vi "UI메시지전달.vi"() -> ()   [LabVIEW 2014]
panel:
  out "에러 출력":errorcluster
  in  "Configuration":T1
  in  "정지":bool
  in  "Stop Control":bool
  in  "Start Control":bool
  in  "Update Configuration":bool
  in  "Connect":bool
  out "메시지 출력":string
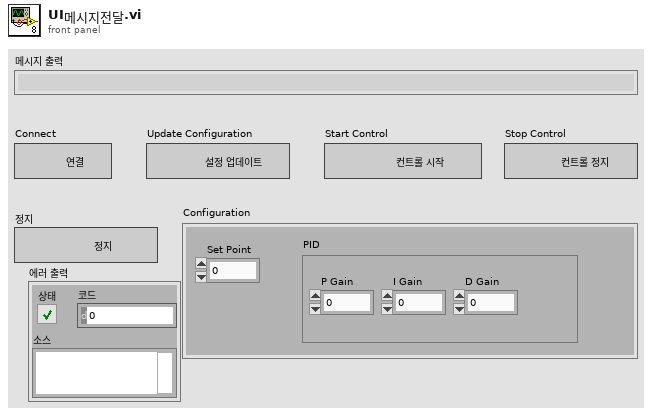
[diagram p1: front panel]
types:
  T1 = cluster{"Set Point":dbl, "PID":cluster{"P Gain":dbl, "I Gain":dbl, "D Gain":dbl}}
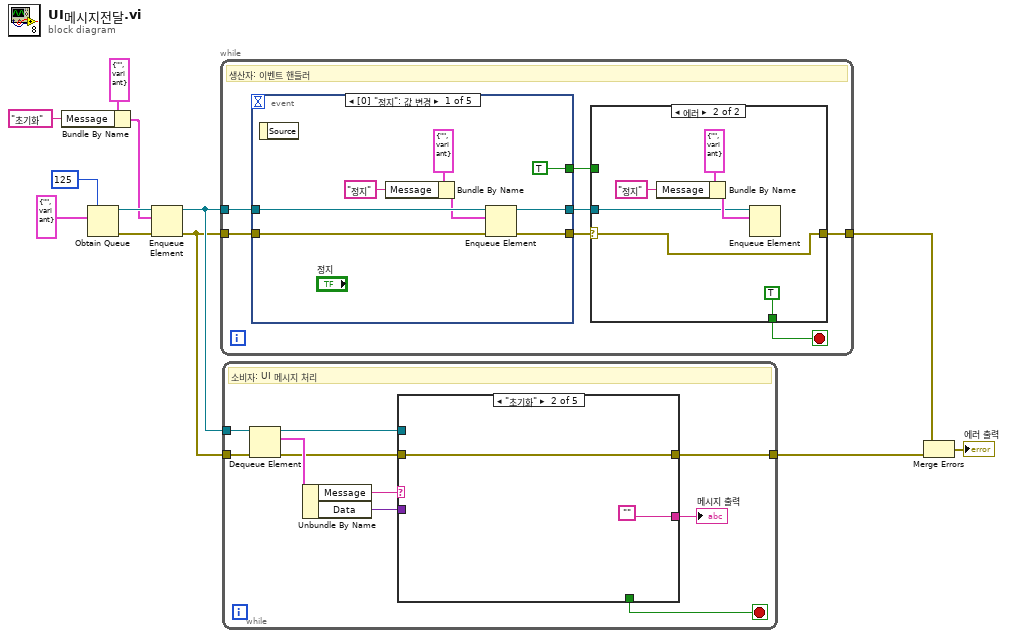
[diagram p0: block diagram]
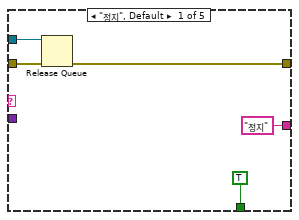
[diagram p2: hidden frame]
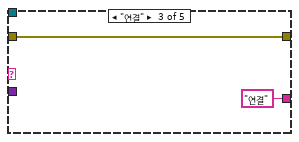
[diagram p3: hidden frame]
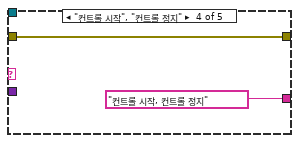
[diagram p4: hidden frame]
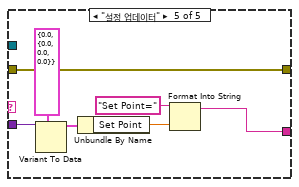
[diagram p5: hidden frame]
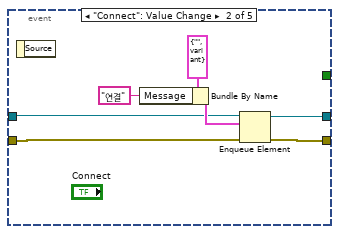
[diagram p7: hidden frame]
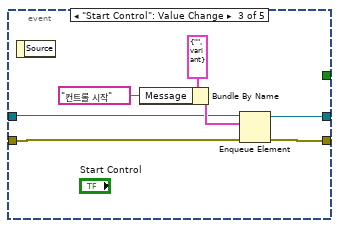
[diagram p8: hidden frame]
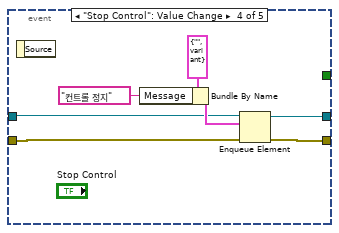
[diagram p9: hidden frame]
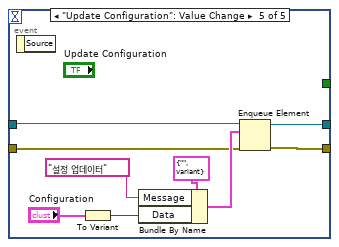
[diagram p10: hidden frame]
diagram:
  n1 = Bundle By Name(cluster=cluster{"Message":string, "Data":variant} {"Message"="", "Data"=variant} ("UI메시지"), "Message"="초기화") -> (w7:cluster{"Message":string, "Data":variant})
  n2 = Obtain Queue(max queue size (-1, unlimited)=125 ("최대 큐 크기(-1,제한없음)"), element data type=cluster{"Message":string, "Data":variant} {"Message"="", "Data"=variant} ("UI메시지")) -> (queue out=w12:refnum<queue>, error out=w11:errorcluster)  [unwired: 3 in, 1 out]
  n3 = Enqueue Element(queue=w12, element=w7, error in (no error)=w11) -> (queue out=w5:refnum<queue>, error out=w4:errorcluster)  [unwired: 1 in, 1 out]
  n4 = while {
    tunnel: w5 -> [w19]
    tunnel: w4 -> [w18]
    tunnel: [w15] -> w3
    stop <- w13 stop-if-true
    # "생산자: 이벤트 핸들러"
    n5 = event shown="[0] \"정지\": 값 변경" {
      selector: _ -> [_ _ _ _ _]
      dyn-events: _ -> [_ _ _ _ _]
      timeout: _ -> [_ _ _ _ _]
      tunnel: w19 -> [w35 w39 w46 w53 w62]
      tunnel: w18 -> [w34 w37 w43 w50 w59]
      tunnel: [w30 w36 w44 w51 w60] -> w17
      tunnel: [w29 w38 w45 w52 w61] -> w16
      tunnel: [TRUE _ _ _ _] -> w14
      event "정지": Value Change {
        n6 = event-data() -> ()  [unwired: 1 in, 1 out]
        n7 = Bundle By Name(cluster=cluster{"Message":string, "Data":variant} {"Message"="", "Data"=variant} ("UI메시지"), "Message"="정지") -> (w31:cluster{"Message":string, "Data":variant})
        n8 = Enqueue Element(queue=w35, element=w31, error in (no error)=w34) -> (queue out=w29:refnum<queue>, error out=w30:errorcluster)  [unwired: 1 in, 1 out]
      }
      event "Connect": Value Change {
        n9 = event-data() -> ()  [unwired: 1 in, 1 out]
        n10 = Bundle By Name(cluster=cluster{"Message":string, "Data":variant} {"Message"="", "Data"=variant} ("UI메시지"), "Message"="연결") -> (w40:cluster{"Message":string, "Data":variant})
        n11 = Enqueue Element(queue=w39, element=w40, error in (no error)=w37) -> (queue out=w38:refnum<queue>, error out=w36:errorcluster)  [unwired: 1 in, 1 out]
      }
      event "Start Control": Value Change {
        n12 = event-data() -> ()  [unwired: 1 in, 1 out]
        n13 = Bundle By Name(cluster=cluster{"Message":string, "Data":variant} {"Message"="", "Data"=variant} ("UI메시지"), "Message"="컨트롤 시작") -> (w47:cluster{"Message":string, "Data":variant})
        n14 = Enqueue Element(queue=w46, element=w47, error in (no error)=w43) -> (queue out=w45:refnum<queue>, error out=w44:errorcluster)  [unwired: 1 in, 1 out]
      }
      event "Stop Control": Value Change {
        n15 = event-data() -> ()  [unwired: 1 in, 1 out]
        n16 = Bundle By Name(cluster=cluster{"Message":string, "Data":variant} {"Message"="", "Data"=variant} ("UI메시지"), "Message"="컨트롤 정지") -> (w54:cluster{"Message":string, "Data":variant})
        n17 = Enqueue Element(queue=w53, element=w54, error in (no error)=w50) -> (queue out=w52:refnum<queue>, error out=w51:errorcluster)  [unwired: 1 in, 1 out]
      }
      event "Update Configuration": Value Change {
        n18 = event-data() -> ()  [unwired: 1 in, 1 out]
        n19 = To Variant(anything="Configuration") -> (Variant=w57:variant)
        n20 = Bundle By Name(cluster=cluster{"Message":string, "Data":variant} {"Message"="", "Data"=variant} ("UI메시지"), "Message"="설정 업데이터", "Data"=w57) -> (w63:cluster{"Message":string, "Data":variant})
        n21 = Enqueue Element(queue=w62, element=w63, error in (no error)=w59) -> (queue out=w61:refnum<queue>, error out=w60:errorcluster)  [unwired: 1 in, 1 out]
      }
    }
    n22 = case shown="에러" w17 {
      selector: w17 -> [w21 w22]
      tunnel: w16 -> [_ w24]
      tunnel: [w21 w22] -> w15
      tunnel: w14 -> [w20 _]
      tunnel: [w20 TRUE] -> w13
      frame No Error {
      }
      frame Error {
        n23 = Bundle By Name(cluster=cluster{"Message":string, "Data":variant} {"Message"="", "Data"=variant} ("UI메시지"), "Message"="정지") -> (w27:cluster{"Message":string, "Data":variant})
        n24 = Enqueue Element(queue=w24, element=w27) -> ()  [unwired: 2 in, 3 out]
      }
    }
  }
  n25 = while {
    tunnel: w5 -> [w75]
    tunnel: w4 -> [w74]
    tunnel: [w68] -> w2
    stop <- w67 stop-if-true
    # "소비자: UI 메시지 처리"
    n26 = Dequeue Element(queue=w75, error in (no error)=w74) -> (queue out=w71:refnum<queue>, element=w73:cluster{"Message":string, "Data":variant}, error out=w70:errorcluster)  [unwired: 1 in, 1 out]
    n27 = Unbundle By Name(w73) -> ("Message"=w72:string, "Data"=w66:variant)
    n28 = case shown="\"초기화\"" w72 {
      tunnel: w71 -> [w80 _ _ _ _]
      tunnel: w70 -> [w79 w81 w84 w86 w93]
      tunnel: ["정지" "" "연결" "컨트롤 시작, 컨트롤 정지" w87] -> w69
      tunnel: [w78 w81 w84 w86 w93] -> w68
      tunnel: [TRUE _ _ _ _] -> w67
      tunnel: w66 -> [_ _ _ _ w92]
      frame "정지", Default {
        n29 = Release Queue(queue=w80, error in (no error)=w79) -> (error out=w78:errorcluster)  [unwired: 1 in, 2 out]
      }
      frame "초기화" {
      }
      frame "연결" {
      }
      frame "컨트롤 시작", "컨트롤 정지" {
      }
      frame "설정 업데이터" {
        n30 = Variant To Data(type=T1 {"Set Point"=0.0, "PID"={"P Gain"=0.0, "I Gain"=0.0, "D Gain"=0.0}} ("Configuration"), Variant=w92) -> (data=w90:T1)  [unwired: 1 in, 1 out]
        n31 = Unbundle By Name(w90) -> ("Set Point"=w89:dbl)
        n32 = Format Into String(initial string="Set Point=" ("초기 문자열"), w89) -> (resulting string=w87:string)  [unwired: 2 in, 1 out]
      }
    }
    "메시지 출력" <- w69
  }
  n33 = Merge Errors(w3, w2) -> (→"에러 출력":errorcluster)
